vi "Destroy LogMeasData Q.vi"(8 "error in (no error)":errorcluster, 10 "wait for activity?":bool) -> (0 "error out":errorcluster, 3 "Final Data":T1[](array[typedef]))   [LabVIEW 2019]
doc: "Developed by Kevin Thompson\nThompson Engineering, LLC\nkevin@thompsonengineering.net"
uses:
  TD MeasData--cluster.ctl
  TD MeasData QRef.ctl
  GBL DataQ Ref.vi
  DataTypes/InverterData--cluster.ctl
  DataTypes/InverterPhaseData--cluster.ctl
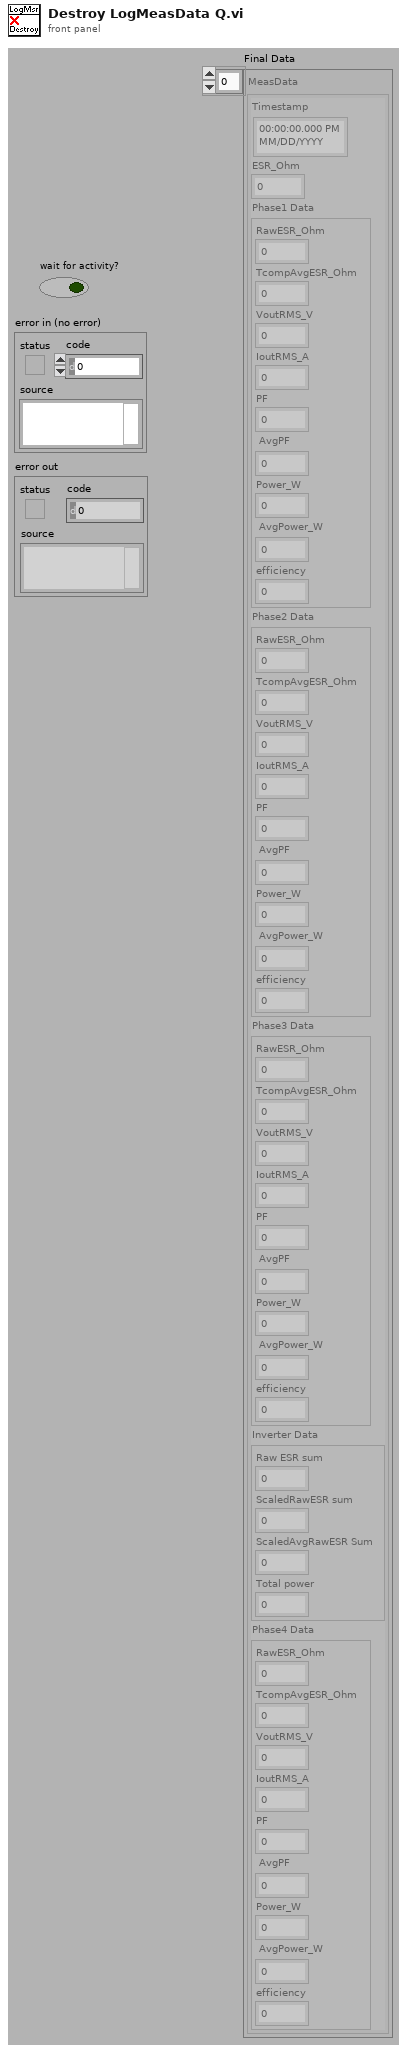
[diagram p1: front panel]
types:
  T1 = typedef "TD MeasData--cluster.ctl" = cluster{"Timestamp":timestamp, "ESR_Ohm":dbl, "Phase1 Data":T2, "Phase2 Data":T2, "Phase3 Data":T2, "Inverter Data":T3, "Phase4 Data":T2}
  T2 = typedef "InverterPhaseData--cluster.ctl" = cluster{"RawESR_Ohm":dbl, "TcompAvgESR_Ohm":dbl, "VoutRMS_V":dbl, "IoutRMS_A":dbl, "PF":dbl, "AvgPF":dbl, "Power_W":dbl, "AvgPower_W":dbl, "efficiency":dbl}
  T3 = typedef "InverterData--cluster.ctl" = cluster{"Raw ESR sum":dbl, "ScaledRawESR sum":dbl, "ScaledAvgRawESR Sum":dbl, "Total power":dbl}
  T4 = typedef "TD MeasData QRef.ctl" = refnum<queue>
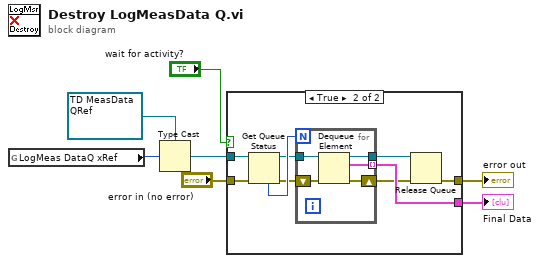
[diagram p0: block diagram]
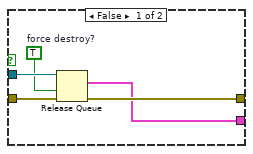
[diagram p2: hidden frame]
diagram:
  n1 = global read "GBL DataQ Ref.vi" "LogMeas DataQ xRef"() -> (w1:u32)
  n2 = Type Cast(type=T4 refnum ("MeasDataQRef"), x=w1) -> (*(type *) &x=w4:T4)
  n3 = case shown="True" "wait for activity?" {
    tunnel: "error in (no error)" -> [w11 w19]
    tunnel: w4 -> [w10 w18]
    tunnel: [w12 w20] -> w6
    tunnel: [w8 w15] -> w3
    frame False {
      w9 = TRUE  # force destroy?
      n4 = Release Queue(queue=w10, force destroy? (F)=w9, error in (no error)=w11) -> (remaining elements=w8:T1[], error out=w12:errorcluster)  [unwired: 1 out]
    }
    frame True {
      n5 = Get Queue Status(queue=w18, error in (no error)=w19) -> (queue out=w14:T4, error out=w16:errorcluster, # elements in queue=w17:i32)  [unwired: 1 in, 5 out]
      n6 = for {
        N: w17 -> [_]
        tunnel: [w26] -> w21
        shift-right: [w23] -> w13
        shift-left: w16 -> [w25]
        tunnel: [w24] -> w15 mode=indexing
        tunnel: w14 -> [w22]
        n7 = Dequeue Element(queue=w22, error in (no error)=w25) -> (queue out=w26:T4, element=w24:T1, error out=w23:errorcluster)  [unwired: 1 in, 1 out]
      }
      n8 = Release Queue(queue=w21, error in (no error)=w13) -> (error out=w20:errorcluster)  [unwired: 1 in, 2 out]
    }
  }
  "error out" <- w6
  "Final Data" <- w3
